vi "CreateSMGR_01_file.vi"(7 "file path to write":path, 8 "error in":errorcluster, 10 "Waveform Graph":waveform(i16)[](graph), 11 "meas_point":i32=4) -> (0 "error out":errorcluster, 1 "microseconds str":string, 2 "date str":string, 3 "file path out":path, 4 "max_values":string[](array[string]))   [LabVIEW 2010]
panel:
  out "dt":dbl format="%#_6f"
  out "max_value str":string
  # "Записываем данные в смешанном виде (текстовый/бинарный)\n-------------------------------------------------------------------------------\nСправка по формату лежит здесь\nhttp://smgr-devel.alwaysdata.net/doku.php?id=start\n\nЕсли включен дебаг, то в файл записываются две синусоиды\nа время ставится текущее"
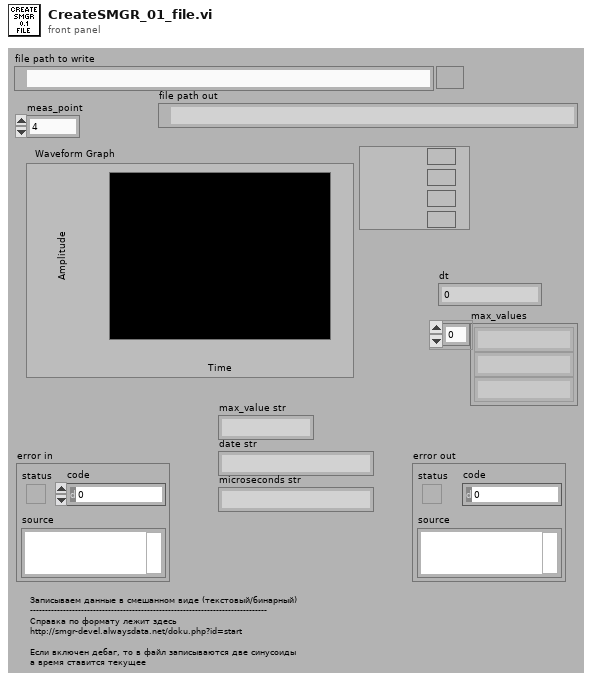
[diagram p1: front panel]
types:
  T1 = enum16{"sync", "phase_a", "phase_b", "phase_c", "ground"}
  T2 = enum16{"big-endian, network order", "native, host order", "little-endian"}
  T3 = enum16{"open", "replace", "create", "open or create", "replace or create", "replace or create with confirmation"}
  T4 = typedef "LVDateTimeRec.ctl" = cluster{"fractional second":dbl, "second":i32, "minute":i32, "hour":i32, "day of month":i32, "month":i32, "year":i32, "day of week":i32, "day of year":i32, "DST":i32}
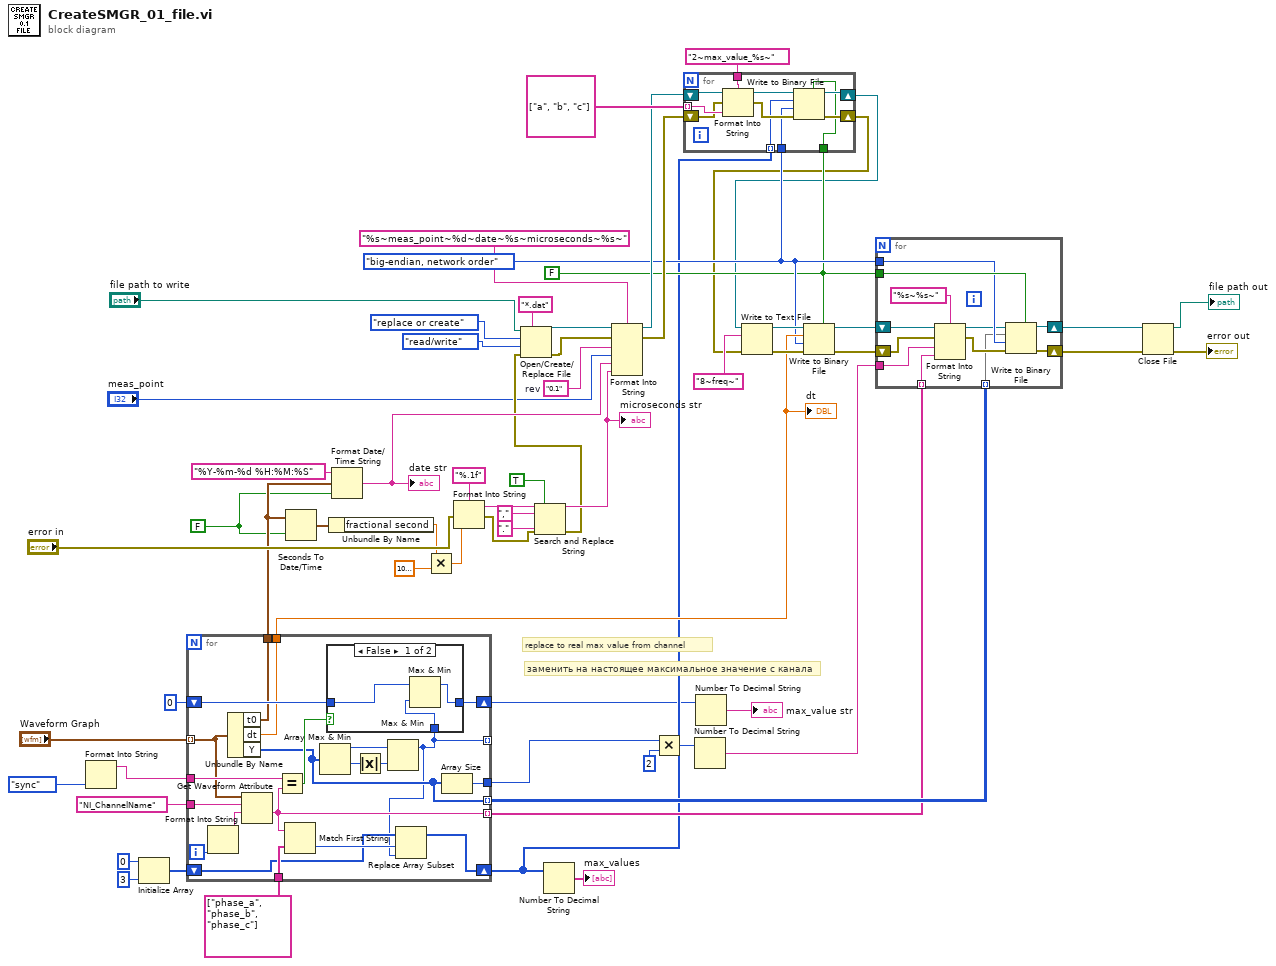
[diagram p0: block diagram]
diagram:
  w17 = FALSE ("to UTC (F)")
  w54 = "0.1"  # rev
  w5 = FALSE ("prepend array or string size? (T)")
  w6 = T2."big-endian, network order" ("byte order (0:big-endian, network order)")
  # "заменить на настоящее максимальное значение с канала"
  # "replace to real max value from channel"
  n1 = Format Into String(T1."sync") -> (resulting string=w24:string)  [unwired: 3 in, 1 out]
  n2 = Initialize Array(i16 0 ("element"), 3 ("dimension size")) -> (w12:i16[])
  n3 = for {
    tunnel: "Waveform Graph" -> [w80] mode=indexing
    tunnel: [w70] -> w47 mode=indexing
    tunnel: [w68] -> w16 mode=indexing
    shift-right: [w81] -> w1
    shift-left: i16 0 -> [w84]
    tunnel: w24 -> [w83]
    tunnel: "NI_ChannelName" -> [w79]
    tunnel: [w76] -> w23
    tunnel: [w75] -> w22
    tunnel: [w74] -> w21
    tunnel: [w64] -> _ mode=indexing
    tunnel: string[] ["phase_a", "phase_b", "phase_c"] -> [w69]
    shift-right: [w65] -> w2
    shift-left: w12 -> [w66]
    i -> [w78]
    n4 = Format Into String(w78) -> (resulting string=w77:string)  [unwired: 3 in, 1 out]
    n5 = Unbundle By Name(w80) -> ("t0"=w75:timestamp, "dt"=w76:dbl, "Y"=w70:i16[])
    n6 = Get Waveform Attribute(5:w77, 6:w79, 7:w80) -> (1:w68:string)  [unwired: 1 in, 3 out]
    n7 = Equal?(x=w83, y=w68) -> (x = y?=w82:bool)
    n8 = Match First String(2:w69, 3:w68) -> (0:w67:i32)  [unwired: 1 out]
    n9 = Array Max & Min(array=w70) -> (max value=w72:i16, min value=w71:i16)  [unwired: 2 out]
    n10 = Absolute Value(x=w71) -> (abs(x)=w73:i16)
    n11 = Max & Min(x=w72, y=w73) -> (max(x,y)=w64:i16)  [unwired: 1 out]
    n12 = case shown="False" w82 {
      tunnel: w84 -> [w86 w88]
      tunnel: [w87 w88] -> w81
      tunnel: w64 -> [w85 _]
      frame False {
        n13 = Max & Min(x=w86, y=w85) -> (max(x,y)=w87:i16)  [unwired: 1 out]
      }
      frame True {
      }
    }
    n14 = Replace Array Subset(array=w66, new element=w64, index=w67) -> (w65:i16[])
    n15 = Array Size(array=w70) -> (size(s)=w74:i32)
  }
  "dt" <- w23
  n16 = Seconds To Date/Time(time stamp (now)=w22, to UTC (F)=w17) -> (date time rec=w56:T4)
  n17 = Unbundle By Name(w56) -> ("fractional second"=w32:dbl)
  n18 = Format Date/Time String(time format string (%c)="%Y-%m-%d %H:%M:%S", seconds (now)=w22, UTC format=w17) -> (date/time string=w53:string)
  "date str" <- w53
  n19 = Multiply(x=w32, y=1000000.0) -> (x*y=w30:dbl)
  n20 = Format Into String(format string="%.1f", error in="error in", w30) -> (resulting string=w41:string, error out=w39:errorcluster)  [unwired: 1 in]
  n21 = Search and Replace String(replace all?=TRUE ("replace all? (F)"), input string=w41, search string=",", replace string="." ("replace string (\"\")"), error in=w39) -> (result string=w35:string, error out=w34:errorcluster)  [unwired: 3 in, 2 out]
  "microseconds str" <- w35
  n22 = Open/Create/Replace File(file path (use dialog)="file path to write", error in=w34, prompt="*.dat", operation (0:open)=T3."replace or create", access (0:read/write)=enum16{"read/write", "read-only", "write-only"}."read/write") -> (refnum out=w59:refnum<file>, error out=w58:errorcluster)  [unwired: 1 in, 1 out]
  n23 = Number To Decimal String(number=w2) -> (decimal integer string=→"max_values":string[])  [unwired: 1 in]
  n24 = Format Into String(format string="%s~meas_point~%d~date~%s~microseconds~%s~", initial string=w59, error in=w58, w54, "meas_point", w53, w35) -> (resulting string=w8:refnum<file>, error out=w7:errorcluster)
  n25 = Multiply(x=w21, y=2 ("index")) -> (x*y=w45:i32)
  n26 = for {
    tunnel: "2~max_value_%s~" ("prompt") -> [w99]
    tunnel: string[] ["a", "b", "c"] -> [w98] mode=indexing
    shift-right: [w96] -> w4
    shift-left: w8 -> [w95]
    shift-right: [w92] -> w3
    shift-left: w7 -> [w94]
    tunnel: w2 -> [w91] mode=indexing
    tunnel: w6 -> [w90]
    tunnel: w5 -> [w89]
    n27 = Format Into String(format string=w99, initial string=w95, error in=w94, w98) -> (resulting string=w97:refnum<file>, error out=w93:errorcluster)
    n28 = Write to Binary File(file (use dialog)=w97, data=w91, error in=w93, 5:w89, 9:w90) -> (refnum out=w96:refnum<file>, error out=w92:errorcluster)  [unwired: 1 in, 1 out]
  }
  n29 = Number To Decimal String(number=w45) -> (decimal integer string=w46:string)  [unwired: 1 in]
  n30 = Number To Decimal String(number=w1) -> (decimal integer string=→"max_value str":string)  [unwired: 1 in]
  n31 = Write to Text File(file (use dialog)=w4, text="8~freq~" ("prompt"), error in=w3) -> (refnum out=w51:refnum<file>, error out=w50:errorcluster)  [unwired: 1 in, 1 out]
  n32 = Write to Binary File(file (use dialog)=w51, data=w23, error in=w50, 5:w5, 9:w6) -> (refnum out=w49:refnum<file>, error out=w48:errorcluster)  [unwired: 1 in, 1 out]
  n33 = for {
    shift-right: [w104] -> w18
    shift-left: w49 -> [w111]
    shift-right: [w106] -> w19
    shift-left: w48 -> [w108]
    tunnel: w47 -> [w100] mode=indexing
    tunnel: w16 -> [w101] mode=indexing
    tunnel: w6 -> [w109]
    tunnel: w5 -> [w110]
    tunnel: w46 -> [w102]
    n34 = Format Into String(format string="%s~%s~" ("prompt"), initial string=w111, error in=w108, w102, w101) -> (resulting string=w105:refnum<file>, error out=w107:errorcluster)
    n35 = Write to Binary File(file (use dialog)=w105, data=w100, error in=w107, 5:w110, 9:w109) -> (refnum out=w104:refnum<file>, error out=w106:errorcluster)  [unwired: 1 in, 1 out]
  }
  n36 = Close File(refnum=w18, error in=w19) -> (path=→"file path out":path, error out=→"error out":errorcluster)
